vi "LSX Get Version Str Info.vi"(8 "error in (no error)":errorcluster, 9 "lMaxLen":i32, 10 "pcVersInfo":string, 11 "lLSID":i32) -> (0 "error out":errorcluster, 2 "pcVersInfo out":string, 3 "function return":i32)   [LabVIEW 2018, in "Tango.lvlib"]
doc: "TANGOAPI int TANGOCALL LSX_GetVersionStrInfo (int lLSID, char *pcVersInfo, int lMaxLen);"
uses:
  Tango.lvlib
  SubVIs/Tango_DLL.dll
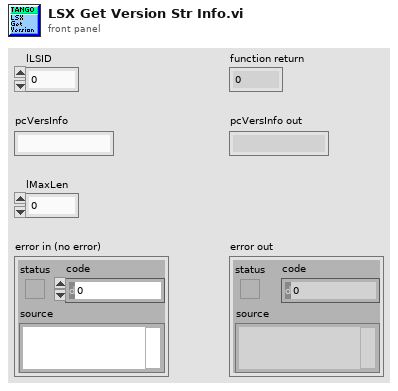
[diagram p1: front panel]
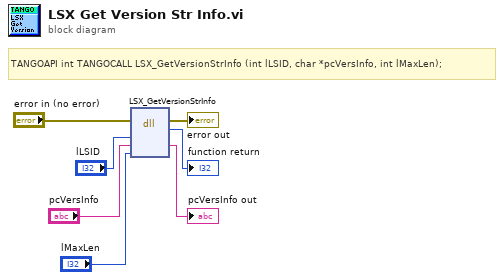
[diagram p0: block diagram]
diagram:
  # "TANGOAPI int TANGOCALL LSX_GetVersionStrInfo (int lLSID, char *pcVersInfo, int lMaxLen);"
  n1 = dll-call lib="C:/Users/Familie/Documents/LabviewIX81/lib/TANGO Stage/SubVIs/Tango_DLL.*" fn="LSX_GetVersionStrInfo"(error in="error in (no error)", "lLSID"="lLSID", "pcVersInfo"="pcVersInfo", "lMaxLen"="lMaxLen") -> (error out=→"error out":errorcluster, →"function return":i32, "pcVersInfo"=→"pcVersInfo out":string)  [unwired: 4 in, 1 out]
